vi "hex divide.vi"() -> ()   [LabVIEW 2020]
panel:
  out "number":u32[](array[numeric]) format="%.0x"
  out "Array":string[](array[string])
  in  "String":string
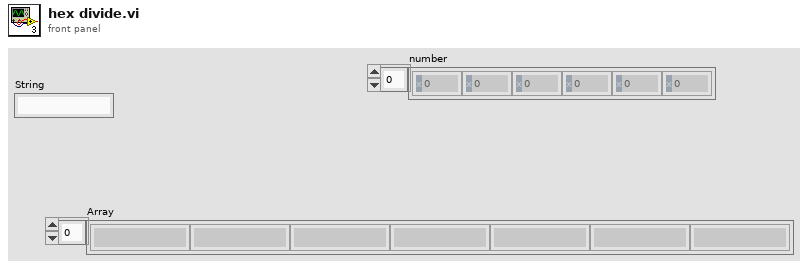
[diagram p1: front panel]
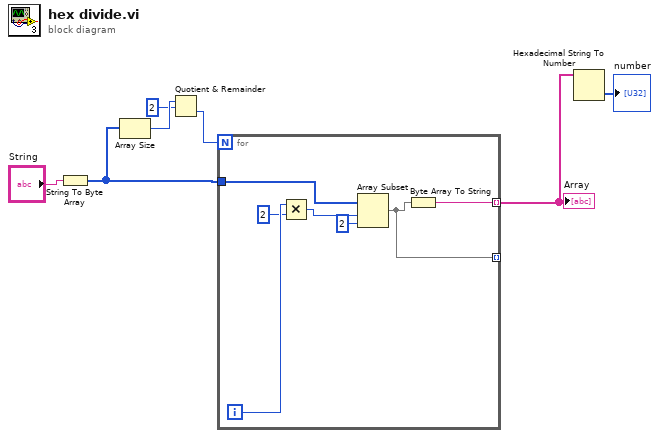
[diagram p0: block diagram]
diagram:
  n1 = String To Byte Array(string="String") -> (unsigned byte array=w6:u8[])
  n2 = Array Size(array=w6) -> (size(s)=w5:i32)
  n3 = Quotient & Remainder(x=w5, y=2) -> (floor(x/y)=w3:i32)  [unwired: 1 out]
  n4 = for {
    N: w3 -> [_]
    tunnel: w6 -> [w14]
    tunnel: [w9] -> w2 mode=indexing
    tunnel: [w8] -> _ mode=indexing
    i -> [w13]
    n5 = Multiply(x=w13, y=2) -> (x*y=w11:i32)
    n6 = Array Subset(array=w14, index=w11, length=2) -> (w8:u8[])
    n7 = Byte Array To String(unsigned byte array=w8) -> (string=w9:string)
  }
  "Array" <- w2
  n8 = Hexadecimal String To Number(string=w2) -> (number=→"number":u32[])  [unwired: 2 in, 1 out]
